vi "abbrevDetectorName.vi"(8 "error in (no error)":errorcluster, 10 "Canonical Name":string, 11 "MatOper in":refnum<class "MatOper.lvclass">) -> (0 "error out":errorcluster, 2 "Abbreviated Detector Name":string, 3 "MatOper out":refnum<class "MatOper.lvclass">)   [LabVIEW 2016, in "OfcFunc.lvlib" / "MatOper.lvclass"]
doc: "Abbreviate the canonical detector name (e.g. \"R:2,2 S:1,1\" to \"R22_S11\")."
uses:
  MatOper.lvclass
  <vilib>/regexp/Match Regular Expression.xnode
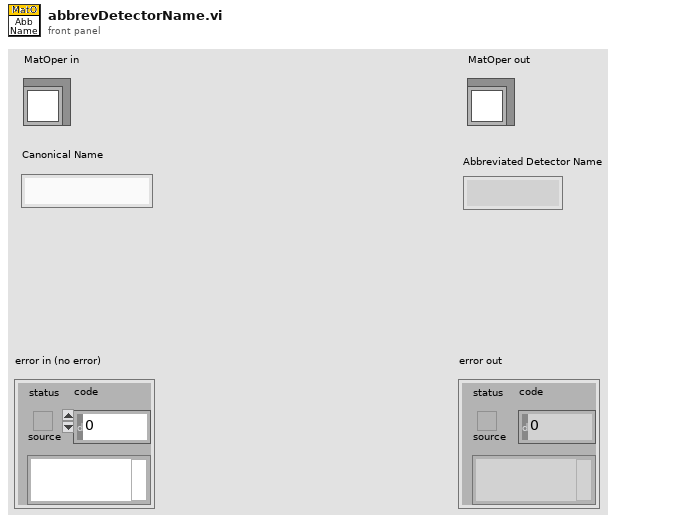
[diagram p1: front panel]
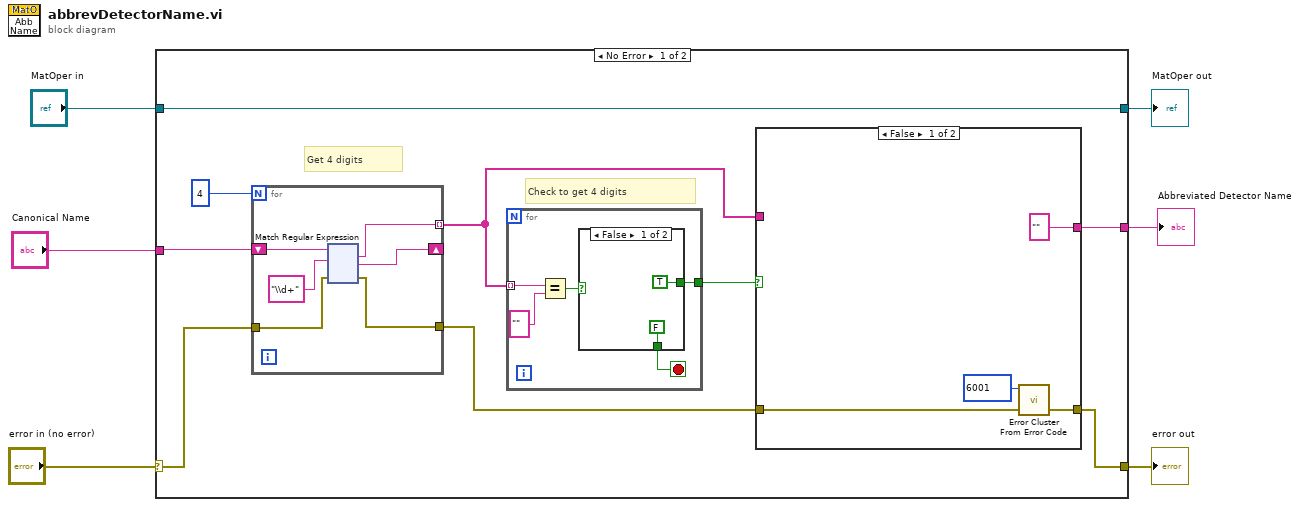
[diagram p0: block diagram]
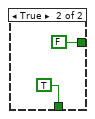
[diagram p2: hidden frame]
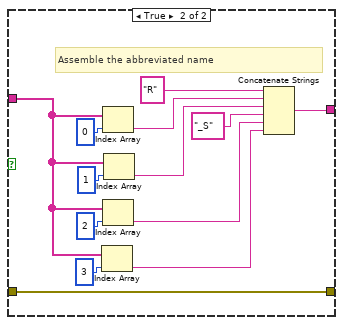
[diagram p3: hidden frame]
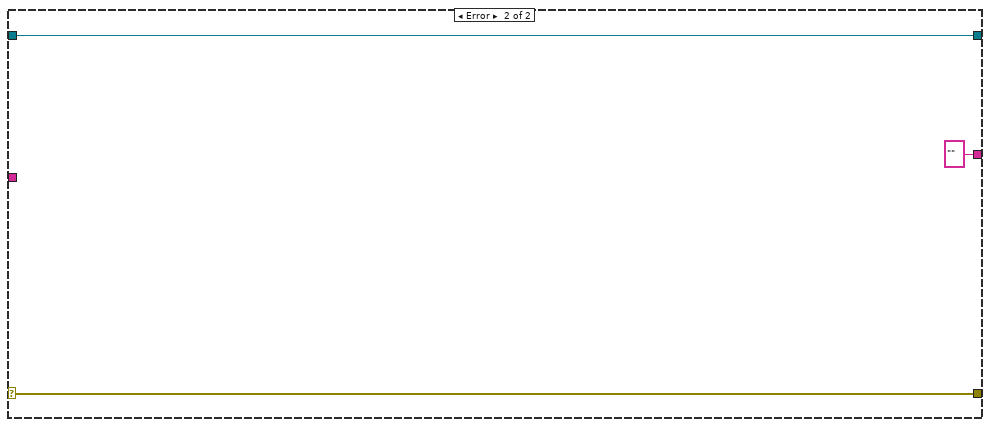
[diagram p4: hidden frame]
diagram:
  n1 = case shown="No Error" "error in (no error)" {
    selector: "error in (no error)" -> [w9 w164]
    tunnel: [w8 w164] -> w5
    tunnel: [w15 w163] -> w3
    tunnel: "MatOper in" -> [w15 w163]
    tunnel: "Canonical Name" -> [w10 _]
    tunnel: [w7 ""] -> w1
    frame No Error {
      # "Check to get 4 digits"
      # "Get 4 digits"
      n2 = for {
        N: 4 -> [_]
        shift-right: [w45] -> _
        shift-left: w10 -> [w47]
        tunnel: [w44] -> w13 mode=indexing
        tunnel: w9 -> [w43]
        tunnel: [w42] -> w11
        n3 = xnode "Match Regular Expression"("input string"=w47, "regular expression"="\\d+", "error in"=w43) -> ("whole match"=w44:string, "after match"=w45:string, "error out"=w42:errorcluster)  [unwired: 3 in, 2 out]
      }
      n4 = for {
        tunnel: w13 -> [w20] mode=indexing
        tunnel: [w17] -> w12
        stop <- w18 stop-if-true
        n5 = Equal?(x=w20, y="") -> (x = y?=w16:bool)
        n6 = case shown="False" w16 {
          tunnel: [FALSE TRUE] -> w18
          tunnel: [TRUE FALSE] -> w17
          frame False {
          }
          frame True {
          }
        }
      }
      n7 = case shown="False" w12 {
        tunnel: ["" w31] -> w7
        tunnel: w13 -> [_ w30]
        tunnel: w11 -> [w25 w29]
        tunnel: [w26 w29] -> w8
        frame False {
          n8 = call <vilib>:"Error Cluster From Error Code.vi"("error in (no error)"=w25, "error code (0)"=6001) -> ("error out"=w26:errorcluster)  [unwired: 7 in]
        }
        frame True {
          # "Assemble the abbreviated name"
          n9 = Index Array(array=w30, index=3) -> (element=w32:string)
          n10 = Index Array(array=w30, index=0) -> (element=w36:string)
          n11 = Index Array(array=w30, index=2) -> (element=w33:string)
          n12 = Index Array(array=w30, index=1) -> (element=w35:string)
          n13 = Concatenate Strings("R" ("string"), w36, w35, "_S" ("string"), w33, w32) -> (w31:string)
        }
      }
    }
    frame Error {
    }
  }
  "error out" <- w5
  "MatOper out" <- w3
  "Abbreviated Detector Name" <- w1
